vi "viewerInitDataVectors.vi"(8 "viewerDataVectors":T2, 10 "Cluster":T1, 11 "viewer.lvclass":refnum<class "viewer.lvclass">) -> (0 "viewerDataVectorsOut":T2, 3 "viewer.lvclassOut":refnum<class "viewer.lvclass">)   [LabVIEW 2011, in "viewer.lvclass"]
uses:
  Pollers/ttm_poller_panel_class/viewer.lvclass
  viewerDataVectors.ctl
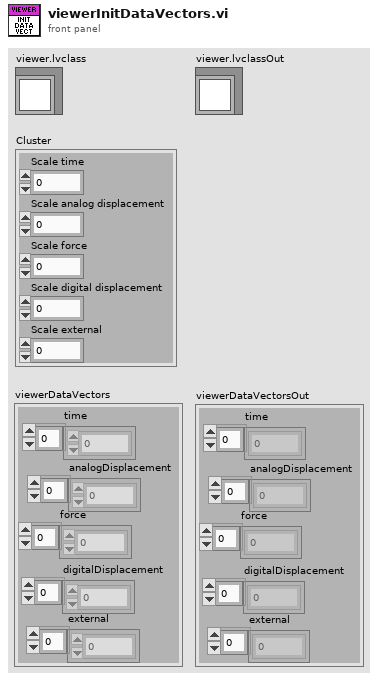
[diagram p1: front panel]
types:
  T1 = cluster{"Scale time":dbl, "Scale analog displacement":dbl, "Scale force":dbl, "Scale digital displacement":dbl, "Scale external":dbl}
  T2 = typedef "viewer.lvclass/viewerDataVectors.ctl" = cluster{"time":dbl[], "analogDisplacement":dbl[], "external":dbl[], "force":dbl[], "digitalDisplacement":dbl[]}
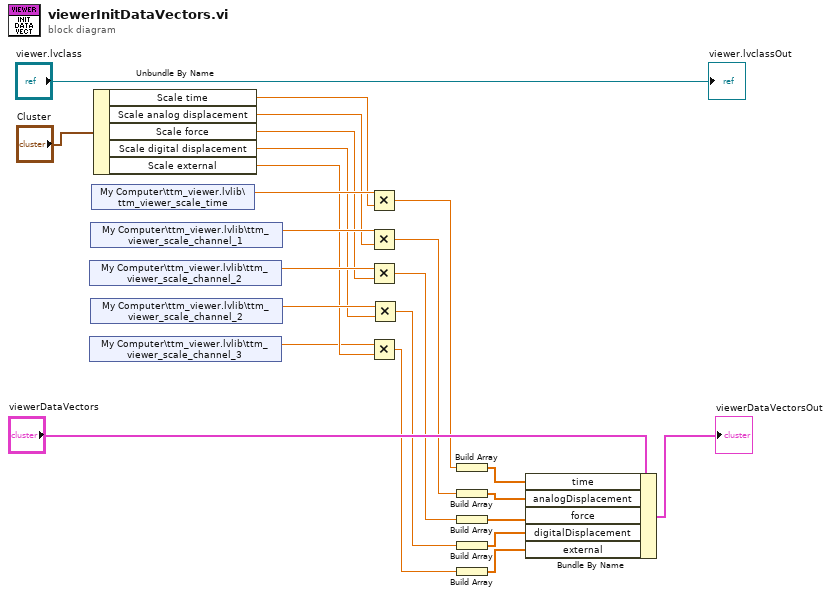
[diagram p0: block diagram]
diagram:
  n1 = shared-variable "My Computer\\ttm_viewer.lvlib\\ttm_viewer_scale_channel_2"() -> (w10:dbl)  [unwired: 1 in, 1 out]
  n2 = shared-variable "My Computer\\ttm_viewer.lvlib\\ttm_viewer_scale_channel_3"() -> (w3:dbl)  [unwired: 1 in, 1 out]
  n3 = shared-variable "My Computer\\ttm_viewer.lvlib\\ttm_viewer_scale_channel_1"() -> (w13:dbl)  [unwired: 1 in, 1 out]
  n4 = shared-variable "My Computer\\ttm_viewer.lvlib\\ttm_viewer_scale_channel_2"() -> (w7:dbl)  [unwired: 1 in, 1 out]
  n5 = shared-variable "My Computer\\ttm_viewer.lvlib\\ttm_viewer_scale_time"() -> (w16:dbl)  [unwired: 1 in, 1 out]
  n6 = Unbundle By Name("Cluster") -> ("Scale time"=w15:dbl, "Scale analog displacement"=w12:dbl, "Scale force"=w9:dbl, "Scale digital displacement"=w5:dbl, "Scale external"=w4:dbl)
  n7 = Multiply(x=w16, y=w15) -> (x*y=w14:dbl)
  n8 = Multiply(x=w13, y=w12) -> (x*y=w11:dbl)
  n9 = Multiply(x=w10, y=w9) -> (x*y=w8:dbl)
  n10 = Multiply(x=w3, y=w4) -> (x*y=w2:dbl)
  n11 = Multiply(x=w7, y=w5) -> (x*y=w6:dbl)
  n12 = Build Array(w14) -> (w22:dbl[])
  n13 = Build Array(w11) -> (w21:dbl[])
  n14 = Build Array(w8) -> (w20:dbl[])
  n15 = Build Array(w6) -> (w19:dbl[])
  n16 = Build Array(w2) -> (w18:dbl[])
  n17 = Bundle By Name(cluster="viewerDataVectors", "time"=w22, "analogDisplacement"=w21, "force"=w20, "digitalDisplacement"=w19, "external"=w18) -> (→"viewerDataVectorsOut":T2)
  "viewer.lvclassOut" <- "viewer.lvclass"
